vi "PH_PSDBController.PC set Exp ID.vi"(0 "i ref in":refnum<vi>, 2 "Exp ID":i16, 5 "error IO":errorcluster) -> (14 "i ref out":refnum<vi>, 19 "error out":errorcluster)   [LabVIEW 2014, in "PH_PSDBController.lvlib"]
doc: "This sets the experiment ID to the GUI and the related DIM service."
uses:
  PH_PSDBController.lvlib
  PH_PSDBWriter/PH_PSDBWriter.Data Status.ctl
  PH_Common/PH_Common.lvlib
  lib.lib/DimLVEvent/LVDimInterface/LVDimInterface.lvlib
  User/Eisenbarth/psdb_lv/PSDB.lvlib
  lib.lib/UtilityLib/UtilityLib.lvlib
  PH_PSDBWriter/PH_PSDBWriter.lvlib
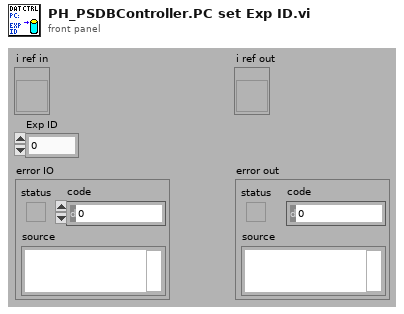
[diagram p1: front panel]
types:
  T1 = typedef "PH_PSDBController.lvlib/PH_PSDBController.i attribute.ctl" = cluster{"GUI Refs":cluster{"Data Status":refnum<vi>, "Current Shot ID":refnum<vi>, "active Subsystems":refnum<vi>, "Experiment Description":refnum<vi>, "Shot Comment":refnum<vi>, "Experiment":refnum<vi>, "Shottype":refnum<vi>, "Sequencer SM State":refnum<vi>, "Instances with Errors":refnum<vi>}, "Service ID Shot ID":i32, "Service ID wanted Subsystem":i32, "Data Status":T2, "Shotinformation":cluster{"Current Experiment ID":i32, "Current Shot Type":i32, "Current Comment":string}, "Data taking?":bool, "Service ID current Shottype":i32, "Service ID current Experiment":i32, "Service ID currentShot Comment":i32, "Service ID possible Shottypes":i32, "Service ID possible Experiments":i32, "possible Experiments":T3[], "possible Shottypes":T3[], "List":cluster{"Info":cluster{"Instance":string, "Data Status":T2}[], "GUI Ref":refnum<vi>, "Classname":string}[], "Subsystems Off?":cluster{"PHELIX_Beamline_fs_YLF_BL_Status":bool, "PHELIX_Beamline_ns_BL_Status":bool, "PHELIX_Beamline_PA_Input_BL_Status":bool, "PHELIX_Beamline_PA_MA_BL_Status":bool, "PHELIX_Beamline_MA_Z6_BL_Status":bool, "PHELIX_Beamline_MA_LB_BL_Status":bool, "PHELIX_Beamline_PA_LL_BL_Status":bool}, "PSDB Credentials":T4}
  T2 = typedef "PH_PSDBWriter.lvlib/PH_PSDBWriter.Data Status.ctl" = i16
  T3 = typedef "PSDB.lvlib/PSDB_Info.ctl" = cluster{"Name":string, "Description":string, "ID":i32}
  T4 = typedef "PH_Common.lvlib/PH_Connection.PSDB Credentials.ctl" = cluster{"PW":string, "ID":string, "DS":string}
  T5 = typedef "NI_Database_API.lvlib/Conn ObjectReference.ctl" = refnum<k1>
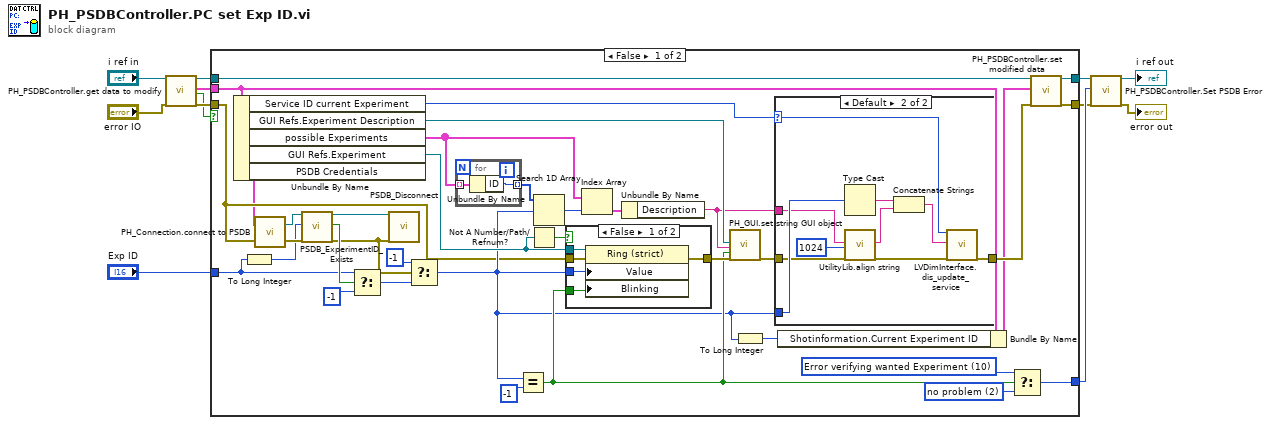
[diagram p0: block diagram]
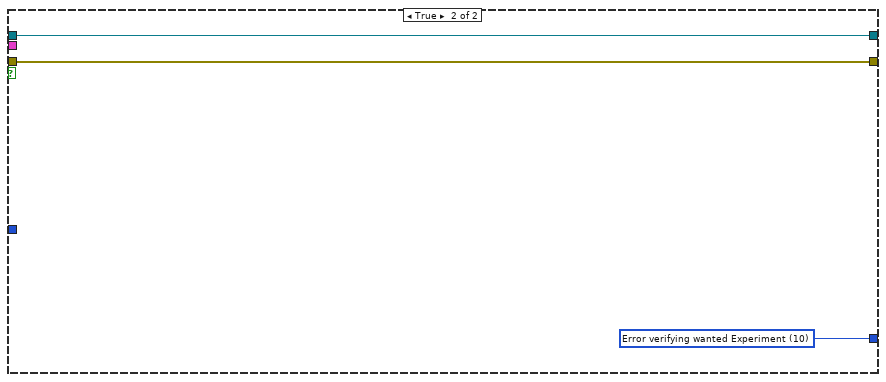
[diagram p4: hidden frame]
diagram:
  n1 = call "PH_PSDBController.get data to modify.vi"("i ref in"="i ref in", "error in (no error)"="error IO") -> ("i ref out"=w3:refnum<vi>, "i attribute"=w12:T1, "timed out"=w1:bool, "error out"=w9:errorcluster)  [unwired: 14 in]
  n2 = case shown="False" w1 {
    tunnel: w12 -> [w16 _]
    tunnel: w9 -> [w15 w69]
    tunnel: "Exp ID" -> [w20 _]
    tunnel: [w27 w68] -> w5
    tunnel: [w24 w69] -> w4
    tunnel: w3 -> [w14 w70]
    tunnel: [w22 w70] -> w2
    frame False {
      w26 = T2 2 items=["no info", "no Data collection", "no problem", "Error getting the instance ID", "Error writing Data to data base", "Error concerning the subsystem", "Error getting the Shot ID", "Error getting the Shot Types", "Error getting the Experiments", "Error verifying wanted Shottype", "Error verifying wanted Experiment"] ("f")
      w28 = T2 10 items=["no info", "no Data collection", "no problem", "Error getting the instance ID", "Error writing Data to data base", "Error concerning the subsystem", "Error getting the Shot ID", "Error getting the Shot Types", "Error getting the Experiments", "Error verifying wanted Shottype", "Error verifying wanted Experiment"] ("Data Status")
      n3 = Unbundle By Name(w16) -> ("Service ID current Experiment"=w41:i32, "GUI Refs.Experiment Description"=w44:refnum<vi>, "possible Experiments"=w33:T3[], "GUI Refs.Experiment"=w42:refnum<vi>, "PSDB Credentials"=w13:T4)
      n4 = To Long Integer(number=w20) -> (32bit integer=w19:i32)
      n5 = call "PH_Connection.connect to PSDB.vi"("error in"=w15, "PSDB Credentials"=w13) -> ("error out"=w38:errorcluster, "connection reference"=w40:T5)
      n6 = call "PSDB_ExperimentID_Exists.vi"("connection reference"=w40, "experiment_id"=w19, "error in (no error)"=w38) -> ("connection reference out"=w39:T5, "id_exists?"=w35:bool, "error out"=w25:errorcluster)  [unwired: 14 in]
      n7 = Select(t=w20, s=w35, f=i16 -1 ("y")) -> (s? t:f=w34:i16)
      n8 = call "PSDB_Disconnect.vi"("connection reference"=w39, "error in (no error)"=w25) -> ()  [unwired: 17 in, 1 out]
      n9 = Select(t=i16 -1, s=w25, f=w34) -> (s? t:f=w17:i16)
      n10 = for {
        tunnel: w33 -> [w50] mode=indexing
        tunnel: [w49] -> w32 mode=indexing
        n11 = Unbundle By Name(w50) -> ("ID"=w49:i32)
      }
      n12 = Equal?(x=w17, y=i16 -1) -> (x = y?=w29:bool)
      n13 = Not A Number/Path/Refnum?(number/path/refnum=w42) -> (NaN/Path/Refnum?=w47:bool)
      n14 = Search 1D Array(1D array=w32, element=w17) -> (index of element=w31:i32)  [unwired: 1 in]
      n15 = case shown="False" w47 {
        tunnel: w15 -> [w55 w56]
        tunnel: [w54 w56] -> w46
        tunnel: w42 -> [w53 _]
        tunnel: w17 -> [w51 _]
        tunnel: w29 -> [w52 _]
        frame False {
          n16 = property class="Ring (strict)"(reference=w53, error in=w55, "Value"=w51, "Blinking"=w52) -> (error out=w54:errorcluster)  [unwired: 1 out]
        }
        frame True {
        }
      }
      n17 = Index Array(array=w33, index=w31) -> (element=w45:T3)
      n18 = Unbundle By Name(w45) -> ("Description"=w30:string)
      n19 = call "PH_GUI.set string GUI object.vi"("GUI object Ref"=w44, "Text"=w30, "Blinking? (false)"=w29, "error in"=w46) -> ("error out"=w48:errorcluster)  [unwired: 15 in]
      n20 = To Long Integer(number=w17) -> (32bit integer=w18:i32)
      n21 = case shown="Default" w41 {
        selector: w41 -> [_ w66]
        tunnel: [w57 w67] -> w23
        tunnel: w48 -> [w57 w61]
        tunnel: w17 -> [_ w65]
        tunnel: w30 -> [_ w59]
        frame -1 {
        }
        frame Default {
          n22 = Type Cast(x=w65) -> (*(type *) &x=w64:string)  [unwired: 1 in]
          n23 = call "UtilityLib.align string.vi"("stringIn"=w59, "stringLength (80)"=u16 1024, "error in (no error)"=w61) -> ("stringOut"=w58:string, "error out"=w60:errorcluster)  [unwired: 15 in]
          n24 = Concatenate Strings(w64, w58) -> (w63:string)
          n25 = call "LVDimInterface.dis_update_service.vi"("my_serviceID"=w66, "data"=w63, "error in (no error)"=w60) -> ("error out"=w67:errorcluster)  [unwired: 14 in, 2 out]
        }
      }
      n26 = Bundle By Name(cluster=w16, "Shotinformation.Current Experiment ID"=w18) -> (w21:T1)
      n27 = Select(t=w28, s=w29, f=w26) -> (s? t:f=w27:T2)
      n28 = call "PH_PSDBController.set modified data.vi"("i ref in"=w14, "i attribute"=w21, "error in (no error)"=w23) -> ("i ref out"=w22:refnum<vi>, "error out"=w24:errorcluster)  [unwired: 15 in]
    }
    frame True {
      w68 = T2 10 items=["no info", "no Data collection", "no problem", "Error getting the instance ID", "Error writing Data to data base", "Error concerning the subsystem", "Error getting the Shot ID", "Error getting the Shot Types", "Error getting the Experiments", "Error verifying wanted Shottype", "Error verifying wanted Experiment"] ("f")
    }
  }
  n29 = call "PH_PSDBController.Set PSDB Error.vi"("i ref in"=w2, "Data Status"=w5, "error in"=w4) -> ("i ref out"=→"i ref out":refnum<vi>, "error out"=→"error out":errorcluster)  [unwired: 15 in]
